vi "AppConstants.vi"() -> (1 "Error Codes":errorcluster[](array[cluster])=[{"status"=TRUE, "code"=6000, "source"="Data directory no found.  App cannot start without this.\nPlease contact administrator immediatly"}, {"status"=TRUE, "code"=6001, "source"="(OmniDriver32.dll not found App cannot start without this.\nPlease contact administrator immediatly) GenerateFilePaths.vi"}, {"status"=TRUE, "code"=6002, "source"="(common32.dll not found App cannot start without this.\nPlease contact administrator immediatly) GenerateFilePaths.vi"}, {"status"=TRUE, "code"=6003, "source"="(TestConfiguration not found Loading defualt values) GenerateFilePaths.vi"}, {"status"=TRUE, "code"=6004, "source"="(EPI_Wafer_Labels.jpg not found App cannot start without this.\nPlease contact administrator immediatly) GenerateFilePaths.vi"}])   [LabVIEW 2012]
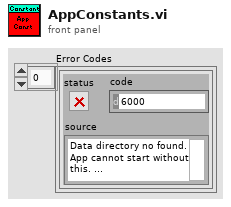
[diagram p1: front panel]
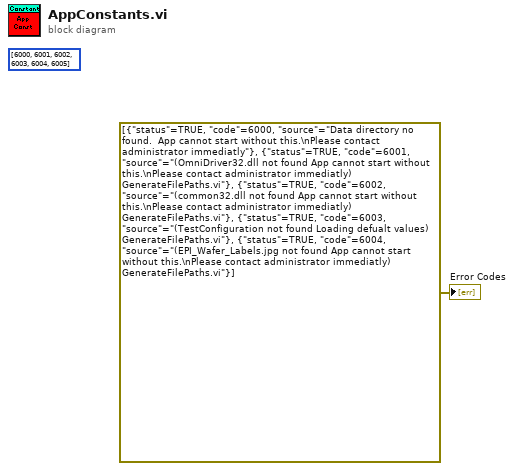
[diagram p0: block diagram]
diagram:
  (unwired) i32[] [6000, 6001, 6002, 6003, 6004, 6005]
  "Error Codes" <- errorcluster[] [{"status"=TRUE, "code"=6000, "source"="Data directory no found.  App cannot start without this.\nPlease contact administrator immediatly"}, {"status"=TRUE, "code"=6001, "source"="(OmniDriver32.dll not found App cannot start without this.\nPlease contact administrator immediatly) GenerateFilePaths.vi"}, {"status"=TRUE, "code"=6002, "source"="(common32.dll not found App cannot start without this.\nPlease contact administrator immediatly) GenerateFilePaths.vi"}, {"status"=TRUE, "code"=6003, "source"="(TestConfiguration not found Loading defualt values) GenerateFilePaths.vi"}, {"status"=TRUE, "code"=6004, "source"="(EPI_Wafer_Labels.jpg not found App cannot start without this.\nPlease contact administrator immediatly) GenerateFilePaths.vi"}] ("appended array")
